vi "Track Nested Model.vi"(8 "error in (no error)":errorcluster, 10 "Nested Model Enqueuer":refnum<class "Message Enqueuer.lvclass">, 11 "IModel in":refnum<class "IModel.lvclass">) -> (0 "error out":errorcluster, 3 "IModel out":refnum<class "IModel.lvclass">)   [LabVIEW 2020, in "MVA Framework.lvlib" / "IModel.lvlib" / "IModel.lvclass"]
doc: "追踪嵌套模型"
uses:
  IModel.lvclass
  <vilib>/ActorFramework/Message Enqueuer/Message Enqueuer.lvclass
  IModel.lvclass/IModel.ctl
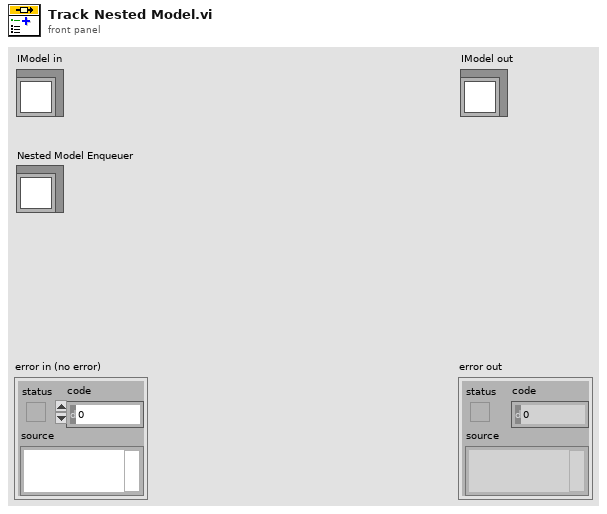
[diagram p1: front panel]
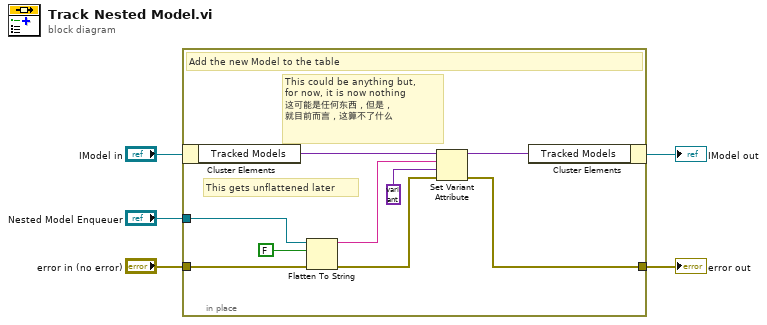
[diagram p0: block diagram]
diagram:
  n1 = in-place {
    in-place-border: "Nested Model Enqueuer" -> [w8]
    in-place-border: "error in (no error)" -> [w12]
    in-place-border: [w7] -> w1
    # "This gets unflattened later"
    # "This could be anything but,\nfor now, it is now nothing\n这可能是任何东西，但是，\n就目前而言，这算不了什么"
    # "Add the new Model to the table"
    n2 = in-place-cluster #1("IModel in") -> ("Tracked Models"=w14:variant)
    n3 = Flatten To String(anything=w8, prepend array or string size? (T)=FALSE, error in (no error)=w12) -> (data string=w9:string, error out=w11:errorcluster)  [unwired: 1 in, 1 out]
    n4 = Set Variant Attribute(Variant=w14, name=w9, value=variant, error in=w11) -> (Variant out=w13:variant, error out=w7:errorcluster)  [unwired: 1 out]
    n5 = in-place-cluster #1("Tracked Models"=w13) -> (→"IModel out":refnum<class "IModel.lvclass">)
  }
  "error out" <- w1
